vi "write_to_excel_v1.vi"(1 "Voltage":dbl format="%#_13g", 2 "First(g), Other(k)":bool, 5 "Illasco SN":string, 6 "error in (no error)":errorcluster, 7 "Test case":string(combo), 8 "Execution Start":timestamp, 9 "Current":dbl format="%#_13g", 10 "Measured value":dbl) -> (0 "error out":errorcluster, 3 "Array 1D":string[](array[string]), 4 "Array 2D":string[][](array[string]))   [LabVIEW 2017]
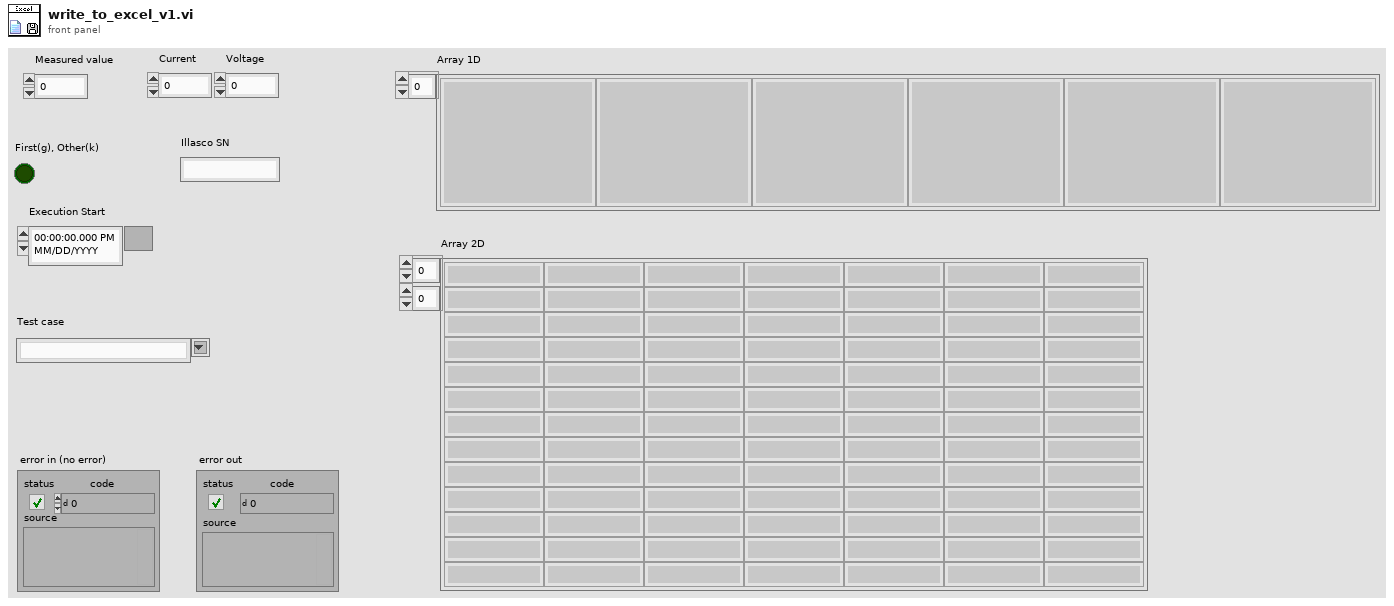
[diagram p1: front panel]
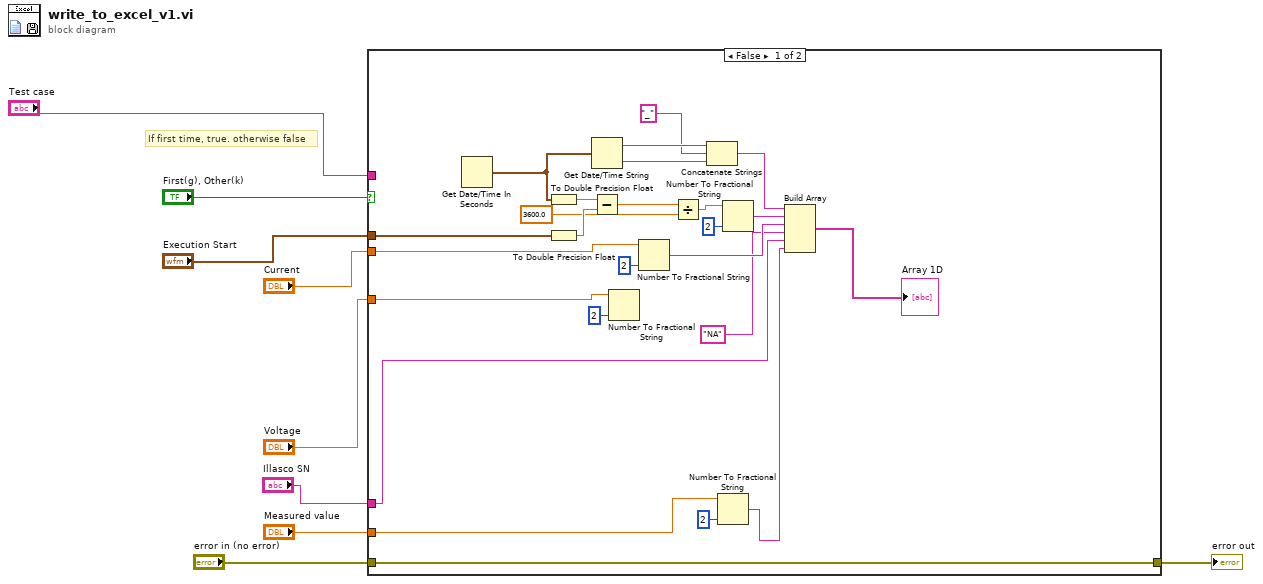
[diagram p0: block diagram]
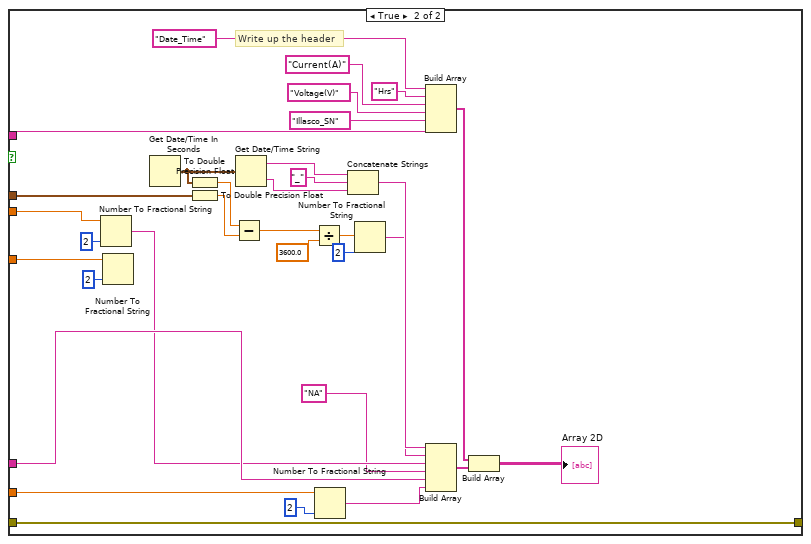
[diagram p2: hidden frame]
diagram:
  # "If first time, true. otherwise false"
  n1 = case shown="False" "First(g), Other(k)" {
    tunnel: "Execution Start" -> [w25 w59]
    tunnel: "Measured value" -> [w13 w37]
    tunnel: "Current" -> [w15 w45]
    tunnel: "Voltage" -> [w10 w43]
    tunnel: "Illasco SN" -> [w24 w50]
    tunnel: "error in (no error)" -> [w22 w48]
    tunnel: [w22 w48] -> w2
    tunnel: "Test case" -> [_ w47]
    frame False {
      n2 = Get Date/Time In Seconds() -> (seconds since 1Jan1904=w27:timestamp)
      n3 = To Double Precision Float(number=w27) -> (double precision float=w30:dbl)
      n4 = To Double Precision Float(number=w25) -> (double precision float=w31:dbl)
      n5 = Get Date/Time String(seconds (now)=w27) -> (date string=w34:string, time string=w33:string)  [unwired: 2 in]
      n6 = Subtract(x=w30, y=w31) -> (x-y=w29:dbl)
      n7 = Number To Fractional String(number=w10, precision (6)=i16 2) -> ()  [unwired: 2 in, 1 out]
      n8 = Number To Fractional String(number=w15, precision (6)=i16 2) -> (F-format string=w14:string)  [unwired: 2 in]
      n9 = Divide(x=w29, y=3600.0) -> (x/y=w17:dbl)
      n10 = Concatenate Strings(w34, "_", w33) -> (w26:string)
      n11 = Number To Fractional String(number=w13, precision (6)=i16 2) -> (F-format string=w12:string)  [unwired: 2 in]
      n12 = Number To Fractional String(number=w17, precision (6)=i16 2) -> (F-format string=w16:string)  [unwired: 2 in]
      n13 = Build Array(w26, w16, w14, "NA" ("element"), w24, w12) -> (→"Array 1D":string[])
    }
    frame True {
      # "Write up the header"
      n14 = Number To Fractional String(number=w45, precision (6)=i16 2) -> (F-format string=w44:string)  [unwired: 2 in]
      n15 = Number To Fractional String(number=w43, precision (6)=i16 2) -> ()  [unwired: 2 in, 1 out]
      n16 = Get Date/Time In Seconds() -> (seconds since 1Jan1904=w60:timestamp)
      n17 = To Double Precision Float(number=w60) -> (double precision float=w63:dbl)
      n18 = To Double Precision Float(number=w59) -> (double precision float=w64:dbl)
      n19 = Subtract(x=w63, y=w64) -> (x-y=w62:dbl)
      n20 = Get Date/Time String(seconds (now)=w60) -> (date string=w67:string, time string=w66:string)  [unwired: 2 in]
      n21 = Divide(x=w62, y=3600.0) -> (x/y=w40:dbl)
      n22 = Number To Fractional String(number=w37, precision (6)=i16 2) -> (F-format string=w36:string)  [unwired: 2 in]
      n23 = Concatenate Strings(w67, "_", w66) -> (w53:string)
      n24 = Number To Fractional String(number=w40, precision (6)=i16 2) -> (F-format string=w42:string)  [unwired: 2 in]
      n25 = Build Array("Date_Time", "Hrs", "Current(A)", "Voltage(V)", "Illasco_SN", w47) -> (w52:string[])
      n26 = Build Array(w53, w42, w44, "NA" ("element"), w50, w36) -> (w51:string[])
      n27 = Build Array(w52, w51) -> (→"Array 2D":string[][])
    }
  }
  "error out" <- w2
